vi "broadcastTiming.vi"(8 "error in (no error)":errorcluster, 10 "Latency in":u32, 11 "DynamicFrameBuilder in":refnum<class "DynamicFrameBuilder.lvclass">) -> (0 "error out":errorcluster, 1 "WaitForRxTimeout":u16, 2 "Latency out":u32, 3 "DynamicFrameBuilder out":refnum<class "DynamicFrameBuilder.lvclass">)   [LabVIEW 2016, in "RTModbus.lvlib" / "DynamicFrameBuilder.lvclass"]
uses:
  DynamicFrameBuilder.lvclass
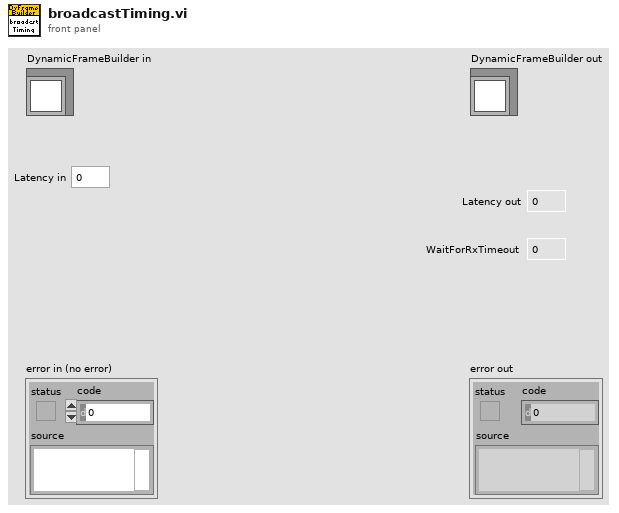
[diagram p1: front panel]
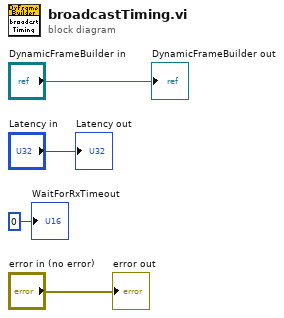
[diagram p0: block diagram]
diagram:
  "error out" <- "error in (no error)"
  "DynamicFrameBuilder out" <- "DynamicFrameBuilder in"
  "WaitForRxTimeout" <- u16 0 ("WaitForRxTimeout")
  "Latency out" <- "Latency in"
